vi "Write Config_CSV_FilePath.vi"(8 "error in (no error)":errorcluster, 10 "Config_CSV_FilePath":path, 11 "MCLB_Template in":refnum<class "SCLB_Template.lvclass">) -> (0 "error out":errorcluster, 3 "MCLB_Template out":refnum<class "SCLB_Template.lvclass">)   [LabVIEW 2021, in "SCLB_Template.lvclass"]
uses:
  SCLB_Template.lvclass
  SCLB_Template.lvclass/SCLB_Template.ctl
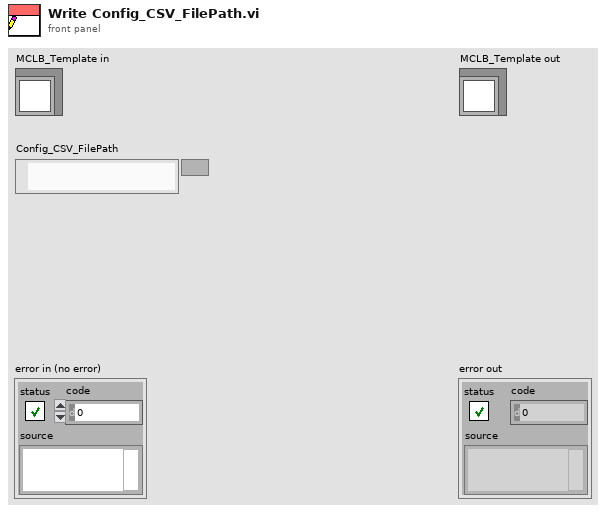
[diagram p1: front panel]
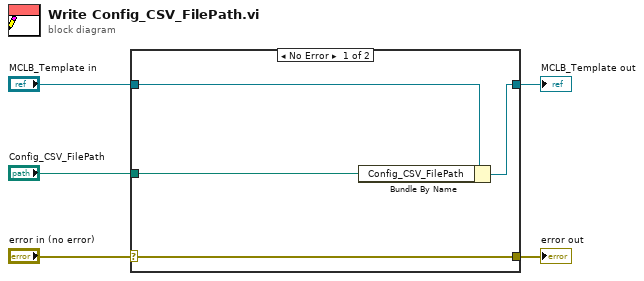
[diagram p0: block diagram]
diagram:
  n1 = case shown="No Error" "error in (no error)" {
    selector: "error in (no error)" -> [w9 w10]
    tunnel: [w9 w10] -> w4
    tunnel: [w7 w11] -> w2
    tunnel: "MCLB_Template in" -> [w8 w11]
    tunnel: "Config_CSV_FilePath" -> [w6 _]
    frame No Error {
      n2 = Bundle By Name(cluster=w8, "Config_CSV_FilePath"=w6) -> (w7:refnum<class "SCLB_Template.lvclass">)
    }
    frame Error {
    }
  }
  "error out" <- w4
  "MCLB_Template out" <- w2
